vi "Build Send.vi"(5 "Target":refnum<vi>, 6 "Class Type":enum16{"Concrete", "Abstract"}(ring), 7 "AppInst":refnum<vi>, 8 "error in (no error)":errorcluster, 9 "Wiring Rules":T1(array[ring]), 10 "Controls":refnum<vi>[](array[refnum]), 11 "Send Method path":path) -> (0 "error out":errorcluster)   [LabVIEW 2020, in "Message Maker.lvlib"]
uses:
  Message Maker.lvlib
  <vilib>/Utility/traverseref.llb/TRef TravTarget.ctl
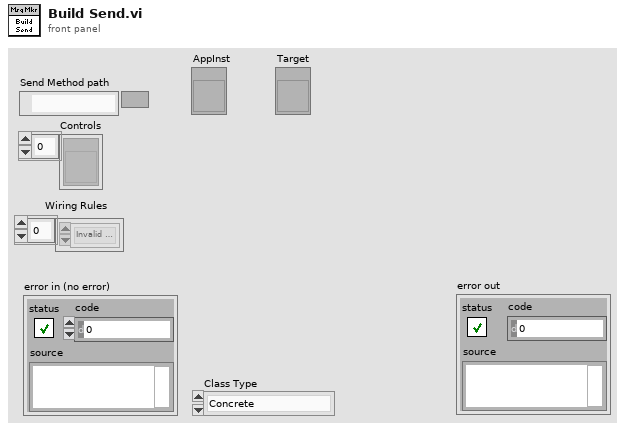
[diagram p1: front panel]
types:
  T1 = enum16{"Invalid Wire Rule", "Required", "Recommended", "Optional", "Dynamic Dispatch"}[]
  T2 = enum32{"Invalid", "Standard", "Closed", "Hidden", "Minimized", "Maximized"}
  T3 = typedef "TRef TravTarget.ctl" = enum16{"FP", "BD", "Other"}
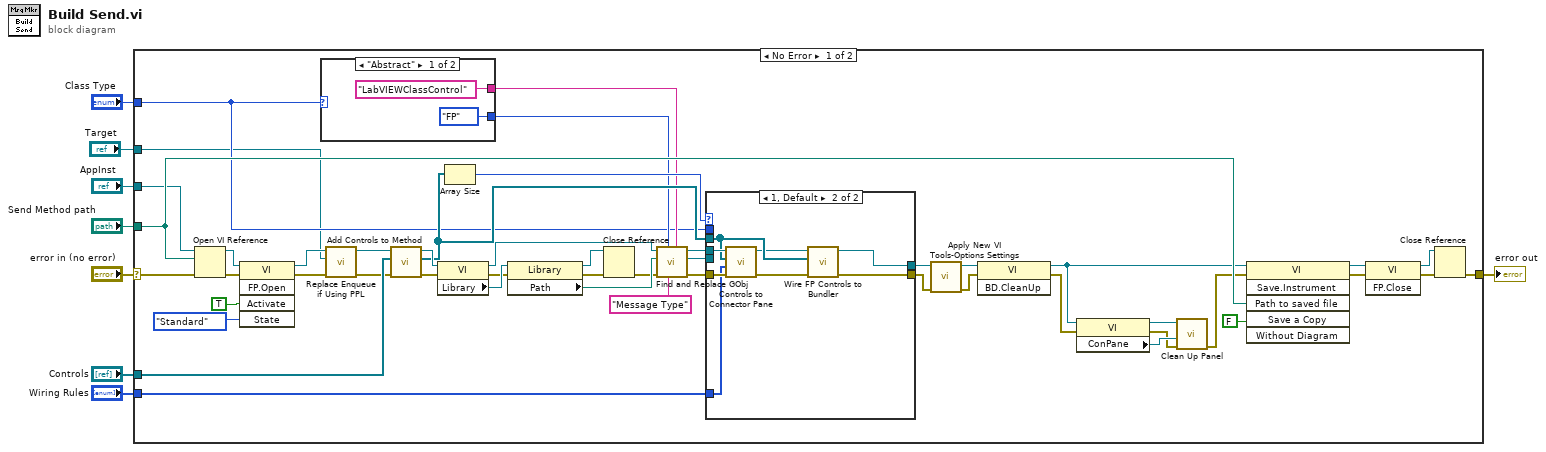
[diagram p0: block diagram]
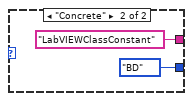
[diagram p2: hidden frame]
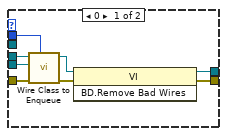
[diagram p3: hidden frame]
diagram:
  n1 = case shown="No Error" "error in (no error)" {
    selector: "error in (no error)" -> [w37 w77]
    tunnel: "Send Method path" -> [w36 _]
    tunnel: [w28 w77] -> w7
    tunnel: "Wiring Rules" -> [w38 _]
    tunnel: "AppInst" -> [w33 _]
    tunnel: "Class Type" -> [w17 _]
    tunnel: "Controls" -> [w14 _]
    tunnel: "Target" -> [w9 _]
    frame No Error {
      n2 = Open VI Reference(application reference (local)=w33, vi path=w36, error in (no error)=w37) -> (vi reference=w41:refnum<vi>, error out=w42:errorcluster)  [unwired: 3 in]
      n3 = invoke class="VI" method="FP.Open"(reference=w41, error in=w42, "Activate"=TRUE ("Activate?"), "State"=T2."Standard") -> (reference out=w10:refnum<vi>, error out=w11:errorcluster)  [unwired: 1 in, 3 out]
      n4 = case shown="\"Abstract\"" w17 {
        tunnel: ["LabVIEWClassControl" ("Class Name") "LabVIEWClassConstant" ("Class Name")] -> w19
        tunnel: [TRef_TravTarget."FP" ("Traverse Target") TRef_TravTarget."BD" ("Traverse Target")] -> w18
        frame "Abstract" {
        }
        frame "Concrete" {
        }
      }
      n5 = call "Replace Enqueue if Using PPL.vi"("error in (no error)"=w11, "Target"=w9, "Send VI ref in"=w10) -> ("error out"=w13:errorcluster, "Send VI ref out"=w12:refnum<vi>)  [unwired: 7 in]
      n6 = call "Add Controls to Method.vi"("error in (no error)"=w13, "Controls in"=w14, "vi ref in"=w12) -> ("error out"=w47:errorcluster, "Controls out"=w45:refnum<vi>[], "vi ref out"=w46:refnum<vi>)  [unwired: 6 in]
      n7 = property class="VI"(reference=w46, error in=w47) -> (reference out=w52:refnum<vi>, error out=w53:errorcluster, "Library"=w54:refnum<vi>)
      n8 = Array Size(array=w45) -> (size(s)=w55:i32)
      n9 = property class="Library"(reference=w54, error in=w53) -> (reference out=w51:refnum<vi>, error out=w50:errorcluster, "Path"=w49:path)
      n10 = Close Reference(reference=w51, error in (no error)=w50) -> (error out=w48:errorcluster)
      n11 = call "Find and Replace GObj.vi"("GObj Class Name"=w19, "GObj Label"="Message Type", "Traverse Target"=w18, "error in (no error)"=w48, "Class Path"=w49, "vi reference in"=w52) -> ("error out"=w35:errorcluster, "Replace"=w16:refnum<vi>, "vi reference out"=w34:refnum<vi>)  [unwired: 3 in]
      n12 = case shown="1, Default" w55 {
        tunnel: [w65 w76] -> w31
        tunnel: [w64 w75] -> w32
        tunnel: w35 -> [w68 w74]
        tunnel: w34 -> [w67 w73]
        tunnel: w45 -> [_ w72]
        tunnel: w38 -> [_ w69]
        tunnel: w17 -> [w62 _]
        tunnel: w16 -> [w61 _]
        frame 0 {
          n13 = call "Wire Class to Enqueue.vi"("Class Type"=w62, "error in (no error)"=w68, "Message Object"=w61, "vi reference"=w67) -> ("error out"=w66:errorcluster, "dup VI Refnum"=w63:refnum<vi>)  [unwired: 6 in]
          n14 = invoke class="VI" method="BD.Remove Bad Wires"(reference=w63, error in=w66) -> (reference out=w64:refnum<vi>, error out=w65:errorcluster)  [unwired: 1 in, 1 out]
        }
        frame 1, Default {
          n15 = call "Controls to Connector Pane.vi"("error in (no error)"=w74, "Wiring Rules"=w69, "Controls"=w72, "vi ref in"=w73) -> ("error out"=w71:errorcluster, "vi ref out"=w70:refnum<vi>)  [unwired: 6 in]
          n16 = call "Wire FP Controls to Bundler.vi"("error in (no error)"=w71, "Controls"=w72, "vi reference in"=w70) -> ("error out"=w76:errorcluster, "vi reference out"=w75:refnum<vi>)  [unwired: 7 in]
        }
      }
      n17 = call <vilib>:"Apply New VI Tools-Options Settings.vi"("error in (no error)"=w31, "VI Refnum"=w32) -> ("error out"=w30:errorcluster, "dup VI Refnum"=w29:refnum<vi>)  [unwired: 8 in]
      n18 = invoke class="VI" method="BD.CleanUp"(reference=w29, error in=w30) -> (reference out=w26:refnum<vi>, error out=w22:errorcluster)  [unwired: 1 in, 1 out]
      n19 = property class="VI"(reference=w26, error in=w22) -> (reference out=w24:refnum<vi>, error out=w23:errorcluster, "ConPane"=w25:refnum<vi>)
      n20 = call "Clean Up Panel.vi"("error in (no error)"=w23, "Conpane"=w25, "VI Refnum"=w24) -> ("error out"=w27:errorcluster)  [unwired: 8 in]
      n21 = invoke class="VI" method="Save.Instrument"(reference=w26, error in=w27, "Path to saved file"=w36, "Save a Copy"=FALSE) -> (reference out=w21:refnum<vi>, error out=w40:errorcluster)  [unwired: 2 in, 4 out]
      n22 = invoke class="VI" method="FP.Close"(reference=w21, error in=w40) -> (reference out=w20:refnum<vi>, error out=w39:errorcluster)  [unwired: 1 in, 1 out]
      n23 = Close Reference(reference=w20, error in (no error)=w39) -> (error out=w28:errorcluster)
    }
    frame Error {
    }
  }
  "error out" <- w7
